vi "Main - ring.vi"() -> ()   [LabVIEW 2024]
doc: "This small application is only a proof of concept. When we have parameters or user data inside an application that could be modified (by the user) at run time, it is important that those changes are 'memorized' when the application is shut down. The next time the application is started it should keep the last configuration made. This is what this application does.\n\nEvery time the user changes the FP data, the changes are saved in the .ini file. If the user closes the application, the FP data is already saved in the .ini configuration file. The next time it is turned on, the data will be loaded again.\n\nIf the user modifies any tag or sector name, or any key name (or its value) in the configuration file (and saves these changes) at run time, the Update button updates this information in the FP of the application, it is the data of the gray fields. This may not be useful in a real application."
uses:
  controls/UI Data.ctl
  controls/string data.ctl
  controls/ring data.ctl
  support/Message Queue/Enqueue Message (Array).vi
  support/Message Queue/Enqueue Message (Single).vi
  dependencies/read-write config ini string data.vi
  <vilib>/Utility/error.llb/Error Cluster From Error Code.vi
  <vilib>/ErrorRing/Error Ring.xnode
  support/Message Queue/Message Queue.lvlib
  support/User Event - Stop/User Event - Stop.lvlib
panel:
  in  "Ring 4":u16(ring) items=["9k", "12k", "18k", "24k"]
  in  "Ring 3":u16(ring) items=["AB ROS", "INVERTER AG", "INVERTER SAMSUNG"]
  in  "Ring 2":u16(ring) items=["MIDEA", "TCL"]
  in  "Ring 1":u16(ring) items=["LOW", "LOW,MID", "LOW,HIGH", "LOW,TURBO", "LOW,MID,HIGH", "LOW,MID,TURBO", "LOW,HIGH,TURBO", "LOW,MID,HIGH,TURBO"]
  out "Display value":string
  in  "Exit":bool
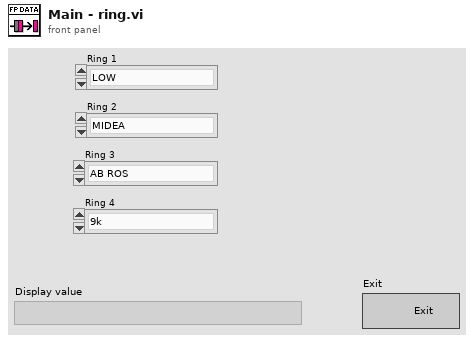
[diagram p1: front panel]
types:
  T1 = typedef "UI Data.ctl" = cluster{"Data Display Ref":refnum<vi>, "Exit Button Ref":refnum<vi>, "user ring data":T2, "ring opts":T2, "Ring Ref":refnum<vi>[], "ring data":T3}
  T2 = typedef "string data.ctl" = cluster{"sectors":string[][], "key names":string[], "values":string[]}
  T3 = typedef "ring data.ctl" = cluster{"option data":string[][]}
  T4 = typedef "Message Queue.lvlib/All Message Queues.ctl" = cluster{"UI":refnum<queue>}
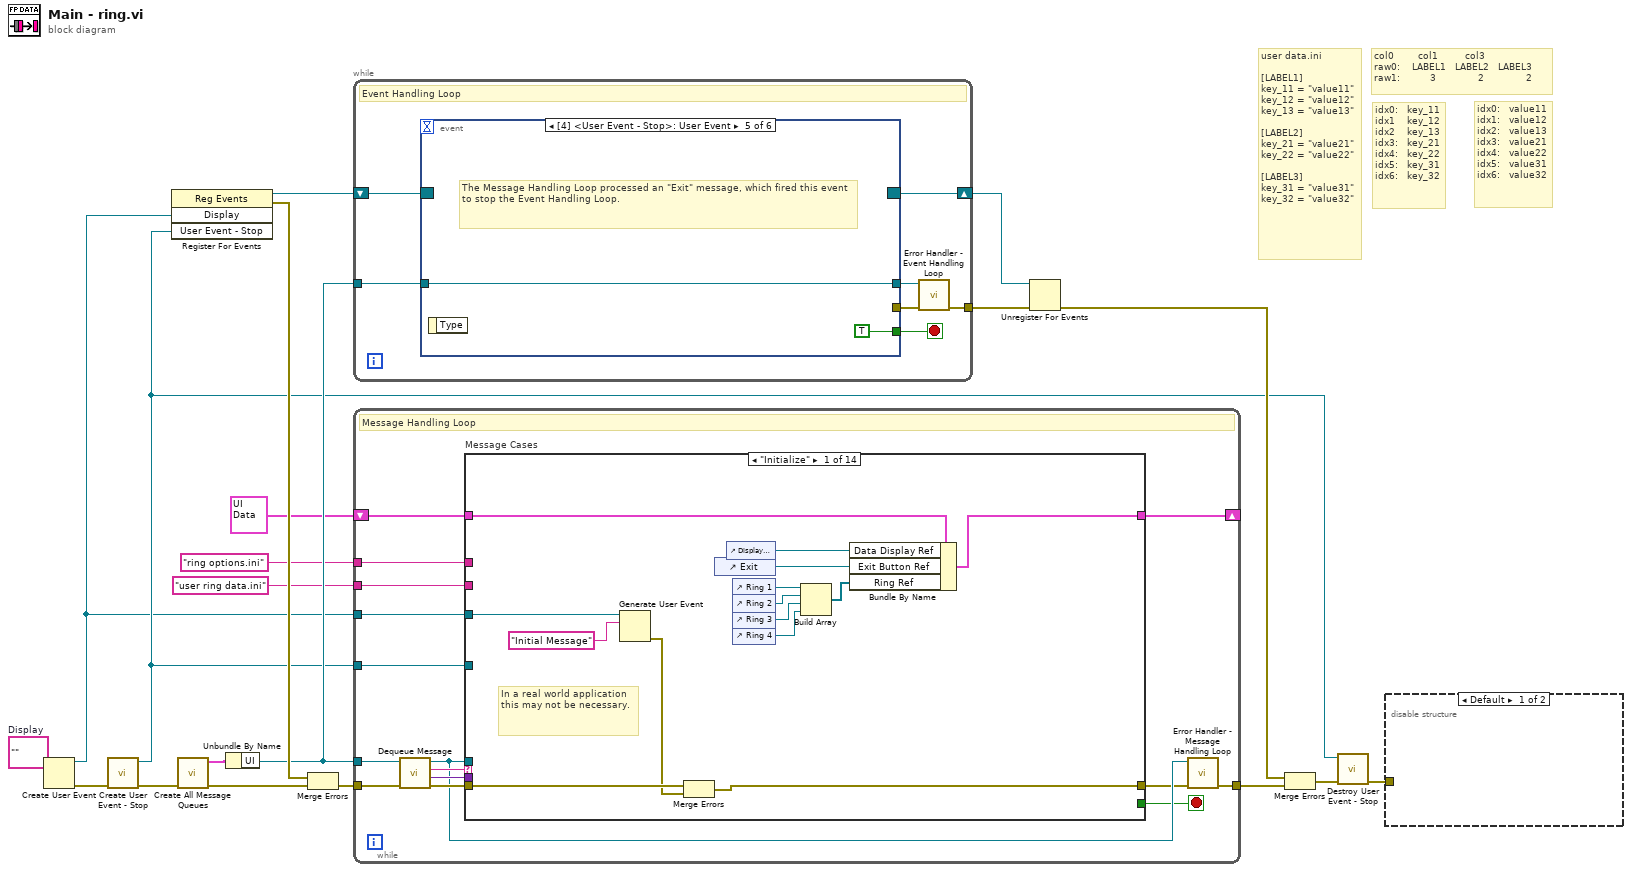
[diagram p0: block diagram]
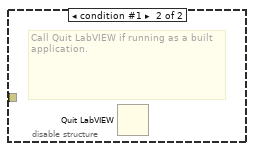
[diagram p2: hidden frame]
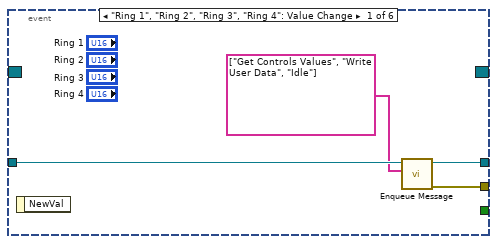
[diagram p3: hidden frame]
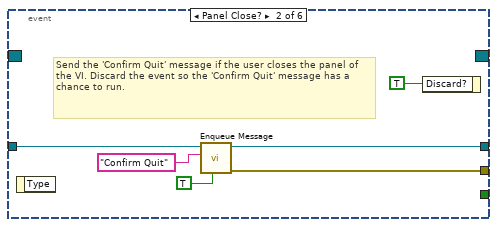
[diagram p4: hidden frame]
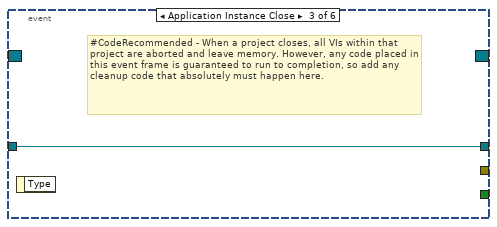
[diagram p5: hidden frame]
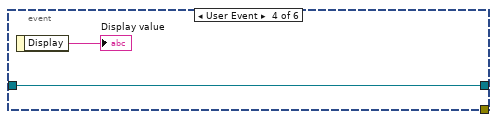
[diagram p6: hidden frame]
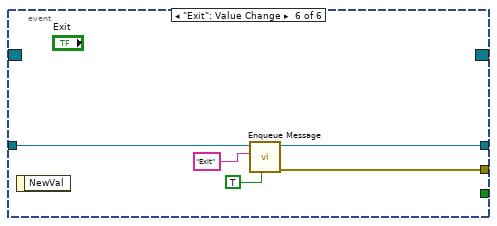
[diagram p7: hidden frame]
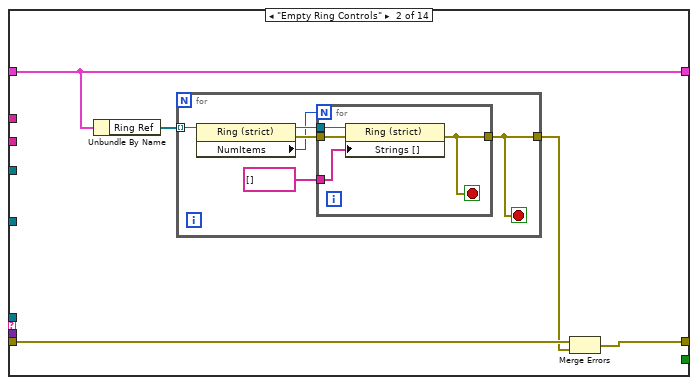
[diagram p8: hidden frame]
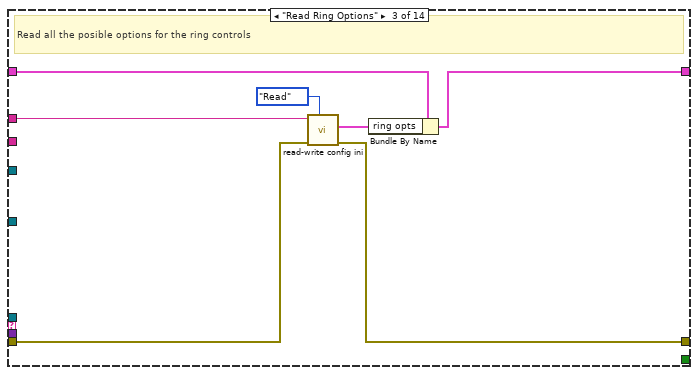
[diagram p9: hidden frame]
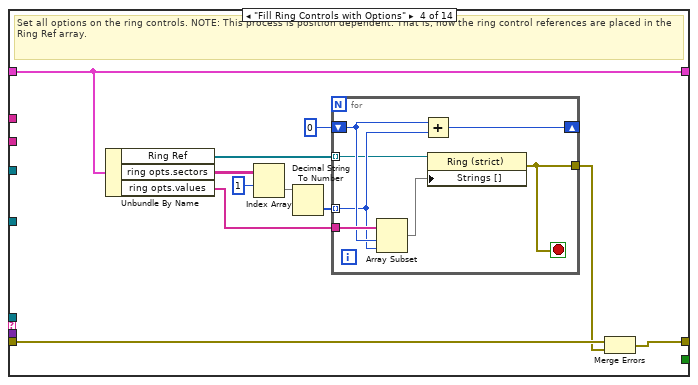
[diagram p10: hidden frame]
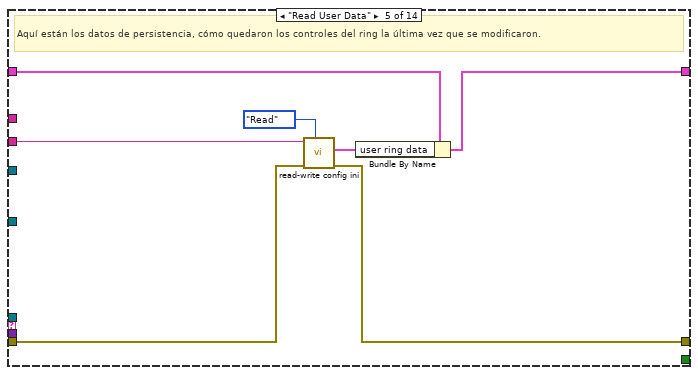
[diagram p11: hidden frame]
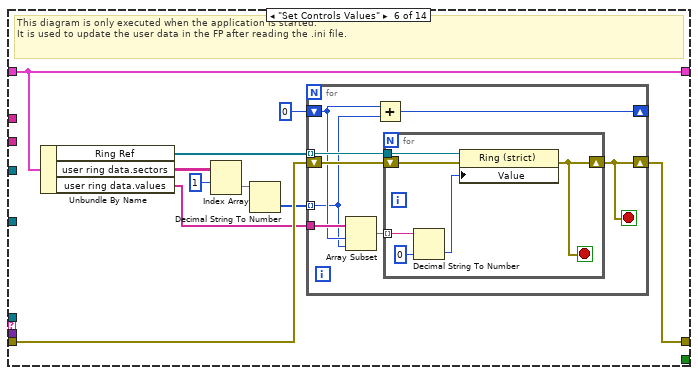
[diagram p12: hidden frame]
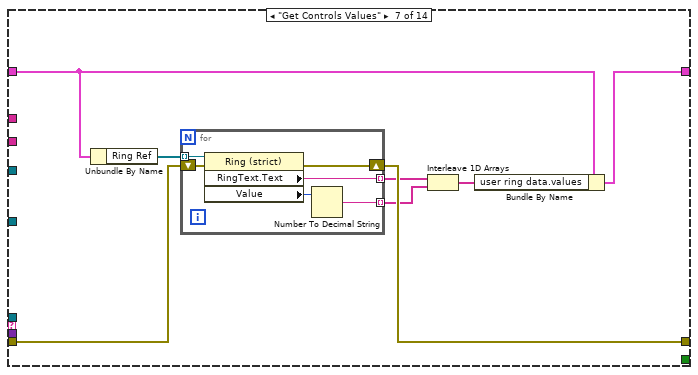
[diagram p13: hidden frame]
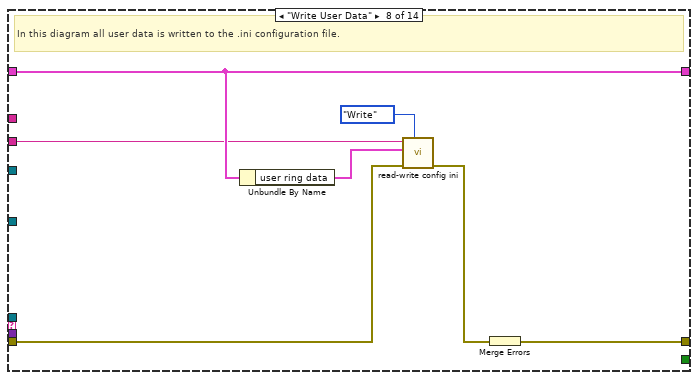
[diagram p14: hidden frame]
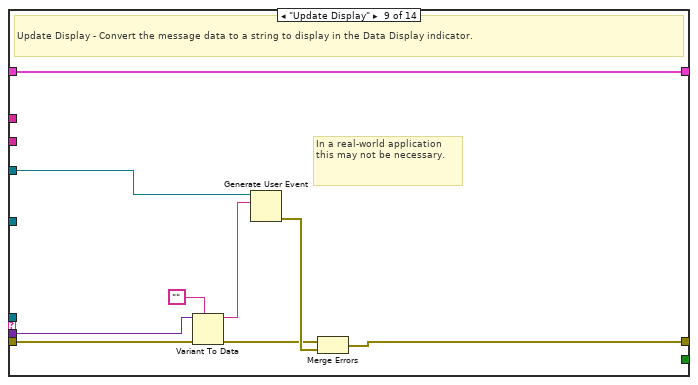
[diagram p15: hidden frame]
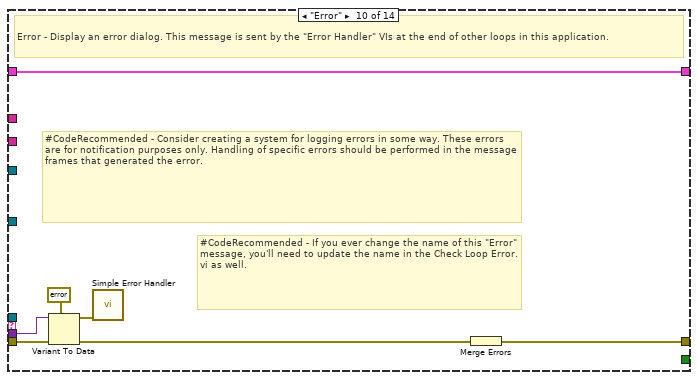
[diagram p16: hidden frame]
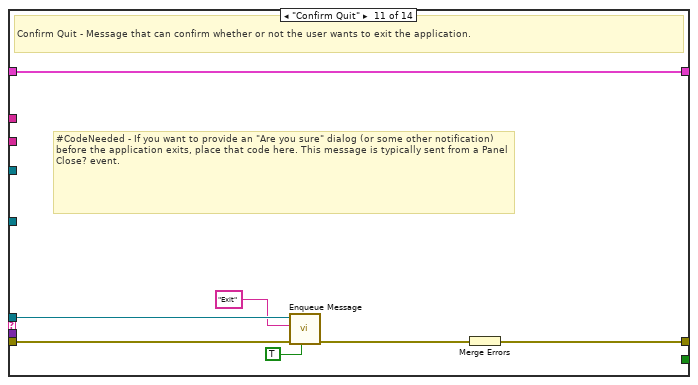
[diagram p17: hidden frame]
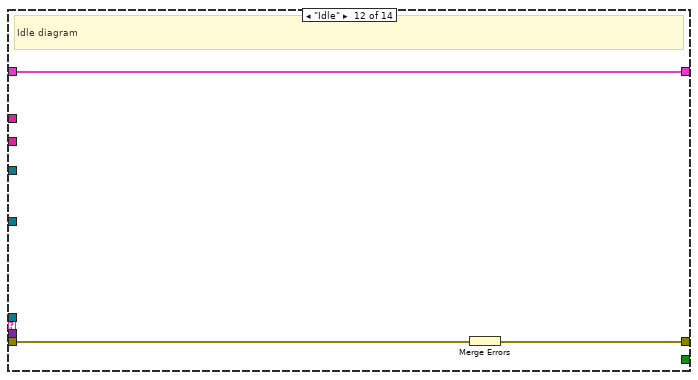
[diagram p18: hidden frame]
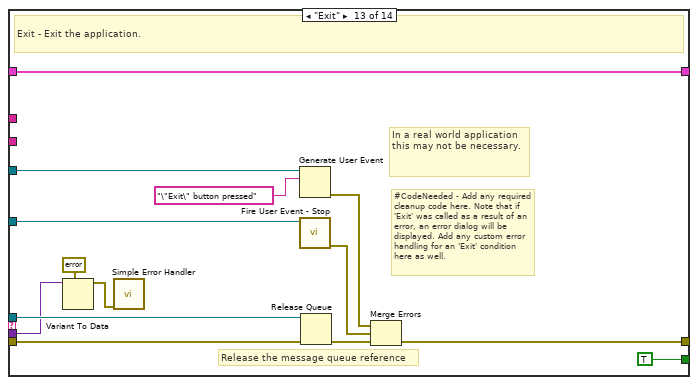
[diagram p19: hidden frame]
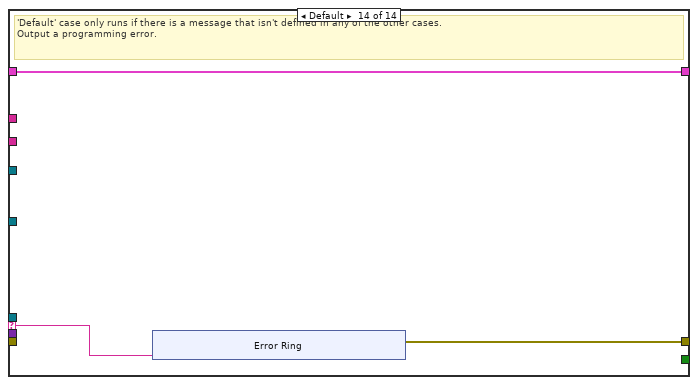
[diagram p20: hidden frame]
diagram:
  w5 = ""  # Display
  # "user data.ini\n\n[LABEL1]\nkey_11 = \"value11\"\nkey_12 = \"value12\"\nkey_13 = \"value13\"\n\n[LABEL2]\nkey_21 = \"value21\"\nkey_22 = \"value22\"\n\n[LABEL3]\nkey_31 = \"value31\"\nkey_32 = \"value32\""
  # "idx0:   value11\nidx1:   value12\nidx2:   value13\nidx3:   value21\nidx4:   value22\nidx5:   value31\nidx6:   value32"
  # "idx0:   key_11\nidx1    key_12\nidx2    key_13\nidx3:   key_21\nidx4:   key_22\nidx5:   key_31\nidx6:   key_32"
  # "col0        col1         col3   \nraw0:    LABEL1   LABEL2   LABEL3\nraw1:          3              2              2"
  n1 = Create User Event(user event datatype=w5) -> (user event=w3:refnum<user-event>, error out=w6:errorcluster)  [unwired: 1 in]
  n2 = call "Create User Event - Stop.vi"("error in (no error)"=w6) -> ("error out"=w15:errorcluster, "User Event - Stop"=w4:refnum<user-event>)  [unwired: 9 in]
  n3 = register-events(w3, w4) -> (reference out=w8:refnum<event-registration>, error out=w20:errorcluster)  [unwired: 2 in]
  n4 = call "Create All Message Queues.vi"("error in (no error)"=w15) -> ("error out"=w19:errorcluster, "Message Queues out"=w18:T4)  [unwired: 9 in]
  n5 = Unbundle By Name(w18) -> ("UI"=w16:refnum<queue>)
  n6 = Merge Errors(w20, w19) -> (w7:errorcluster)
  n7 = while {
    tunnel: w16 -> [w27]
    shift-right: [w25] -> w12
    shift-left: w8 -> [w26]
    tunnel: [w21] -> w9
    stop <- w23 stop-if-true
    # "Event Handling Loop"
    n8 = event shown="[4] <User Event - Stop>: User Event" {
      selector: w26 -> [_ _ _ _ _ _]
      dyn-events: [_ _ _ _ _ _] -> w25
      timeout: _ -> [_ _ _ _ _ _]
      tunnel: [_ _ _ _ TRUE ("Discard?") _] -> w23
      tunnel: w27 -> [w31 w36 w38 w40 w42 w47]
      tunnel: [w29 w35 _ _ _ w46] -> w24
      tunnel: [w30 w34 w38 w40 w42 w45] -> w22
      event "Ring 1", "Ring 2", "Ring 3", "Ring 4": Value Change {
        n9 = event-data() -> ()  [unwired: 1 in, 1 out]
        n10 = call-poly "Enqueue Message.vi"("Message Array"=string[] ["Get Controls Values", "Write User Data", "Idle"], "Message Queue"=w31) -> ("error out"=w29:errorcluster, "dup Message Queue"=w30:refnum<queue>)  [unwired: 8 in]
      }
      event Panel Close? {
        # "Send the 'Confirm Quit' message if the user closes the panel of the VI. Discard the event so the 'Confirm Quit' message has a chance to run."
        n11 = event-data() -> ()  [unwired: 1 in, 1 out]
        n12 = call-poly "Enqueue Message.vi"("Priority Message? (F)"=TRUE, "Message"="Confirm Quit", "Message Queue"=w36) -> ("error out"=w35:errorcluster, "dup Message Queue"=w34:refnum<queue>)  [unwired: 7 in]
        n13 = event-data("Discard?"=TRUE) -> ()  [unwired: 1 in, 1 out]
      }
      event Application Instance Close {
        # "#CodeRecommended - When a project closes, all VIs within that project are aborted and leave memory. However, any code placed in this event frame is guaranteed to run to completion, so add any cleanup code that absolutely must happen here."
        n14 = event-data() -> ()  [unwired: 1 in, 1 out]
      }
      event User Event {
        n15 = event-data() -> ("Display"=→"Display value":string)  [unwired: 1 in]
      }
      event User Event {
        # "The Message Handling Loop processed an \"Exit\" message, which fired this event to stop the Event Handling Loop."
        n16 = event-data() -> ()  [unwired: 1 in, 1 out]
      }
      event "Exit": Value Change {
        n17 = event-data() -> ()  [unwired: 1 in, 1 out]
        n18 = call-poly "Enqueue Message.vi"("Priority Message? (F)"=TRUE, "Message"="Exit", "Message Queue"=w47) -> ("error out"=w46:errorcluster, "dup Message Queue"=w45:refnum<queue>)  [unwired: 7 in]
      }
    }
    n19 = call "Error Handler - Event Handling Loop.vi"("error in (no error)"=w24, "Message Queue"=w22) -> ("dup error in"=w21:errorcluster)  [unwired: 8 in, 1 out]
  }
  n20 = while {
    tunnel: w16 -> [w56]
    shift-right: [w51] -> _
    shift-left: T1 {"Data Display Ref"=refnum, "Exit Button Ref"=refnum, "user ring data"={"sectors"=[], "key names"=[], "values"=[]}, "ring opts"={"sectors"=[], "key names"=[], "values"=[]}, "Ring Ref"=[], "ring data"={"option data"=[]}} ("Data Cluster") -> [w62]
    tunnel: w4 -> [w61]
    tunnel: w7 -> [w60]
    tunnel: [w54] -> w17
    tunnel: w3 -> [w52]
    tunnel: "user ring data.ini" -> [w50]
    tunnel: "ring options.ini" -> [w48]
    stop <- w49 stop-if-true
    # "Message Handling Loop"
    n21 = call "Dequeue Message.vi"("error in (no error)"=w60, "Message Queue"=w56) -> ("error out"=w59:errorcluster, "Message Data"=w57:variant, "Message"=w58:string, "dup Message Queue"=w55:refnum<queue>)  [unwired: 6 in]
    n22 = case "Message Cases" shown="\"Initialize\"" w58 {
      selector: w58 -> [_ _ _ _ _ _ _ _ _ _ _ _ _ w209]
      tunnel: w55 -> [_ _ _ _ _ _ _ _ _ _ w187 _ w208 _]
      tunnel: w59 -> [w72 w81 w96 w109 w119 w133 w154 w162 w172 w184 w191 w194 w201 _]
      tunnel: [w69 w78 w95 w100 w118 w124 w153 w163 w176 w178 w189 w192 w204 w210] -> w53
      tunnel: w62 -> [w76 w80 w94 w108 w123 w132 w150 w168 w177 w183 w190 w193 w207 w211]
      tunnel: [w75 w80 w92 w108 w122 w132 w148 w168 w177 w183 w190 w193 w207 w211] -> w51
      tunnel: [_ _ _ _ _ _ _ _ _ _ _ _ TRUE _] -> w49
      tunnel: w57 -> [_ _ _ _ _ _ _ _ w173 w182 _ _ w198 _]
      tunnel: w61 -> [_ _ _ _ _ _ _ _ _ _ _ _ w203 _]
      tunnel: w52 -> [w71 _ _ _ _ _ _ _ w175 _ _ _ w196 _]
      tunnel: w50 -> [_ _ _ _ w121 _ _ w167 _ _ _ _ _ _]
      tunnel: w48 -> [_ _ w98 _ _ _ _ _ _ _ _ _ _ _]
      frame "Initialize" {
        # "In a real world application this may not be necessary."
        n23 = Generate User Event(user event=w71, event data cluster="Initial Message" ("Initial Message")) -> (error out=w68:errorcluster)  [unwired: 2 in, 1 out]
        n24 = Merge Errors(w72, w68) -> (w69:errorcluster)
        n25 = control-ref of="Exit"() -> (w73:refnum<vi>)
        n26 = control-ref of="Display value"() -> (w74:refnum<vi>)
        n27 = control-ref of="Ring 1"() -> (w67:refnum<vi>)
        n28 = control-ref of="Ring 2"() -> (w66:refnum<vi>)
        n29 = control-ref of="Ring 3"() -> (w65:refnum<vi>)
        n30 = control-ref of="Ring 4"() -> (w64:refnum<vi>)
        n31 = Build Array(w67, w66, w65, w64) -> (w63:refnum<vi>[])
        n32 = Bundle By Name(cluster=w76, "Data Display Ref"=w74, "Exit Button Ref"=w73, "Ring Ref"=w63) -> (w75:T1)
      }
      frame "Empty Ring Controls" {
        n33 = Unbundle By Name(w80) -> ("Ring Ref"=w79:refnum<vi>[])
        n34 = for {
          tunnel: w79 -> [w86] mode=indexing
          tunnel: [w87] -> w77
          stop <- w87 stop-if-true
          n35 = property class="Ring (strict)"(reference=w86) -> (reference out=w85:refnum<vi>, error out=w84:errorcluster, "NumItems"=w83:u32)  [unwired: 1 in]
          n36 = for {
            N: w83 -> [_]
            tunnel: [w91] -> w87
            tunnel: w85 -> [w90]
            tunnel: w84 -> [w89]
            tunnel: string[] [] -> [w88]
            stop <- w91 stop-if-true
            n37 = property class="Ring (strict)"(reference=w90, error in=w89, "Strings []"=w88) -> (error out=w91:errorcluster)  [unwired: 1 out]
          }
        }
        n38 = Merge Errors(w81, w77) -> (w78:errorcluster)
      }
      frame "Read Ring Options" {
        # "Read all the posible options for the ring controls"
        n39 = call-poly "read-write config ini.vi"("Function"=enum16{"Read", "Write"}."Read", "error in (no error)"=w96, "file name"=w98) -> ("error out"=w95:errorcluster, "user data out"=w93:T2)  [unwired: 7 in]
        n40 = Bundle By Name(cluster=w94, "ring opts"=w93) -> (w92:T1)
      }
      frame "Fill Ring Controls with Options" {
        # "Set all options on the ring controls. NOTE: This process is position dependent. That is, how the ring control references are placed in the Ring Ref array."
        n41 = Unbundle By Name(w108) -> ("Ring Ref"=w101:refnum<vi>[], "ring opts.sectors"=w107:string[][], "ring opts.values"=w102:string[])
        n42 = Index Array(array=w107, index (row)=1) -> (element=w105:string[])  [unwired: 1 in]
        n43 = Decimal String To Number(string=w105) -> (number=w104:i32[])  [unwired: 2 in, 1 out]
        n44 = for {
          tunnel: w104 -> [w113] mode=indexing
          shift-right: [w116] -> _
          shift-left: 0 -> [w114]
          tunnel: w102 -> [w115]
          tunnel: w101 -> [w112] mode=indexing
          tunnel: [w110] -> w99
          stop <- w110 stop-if-true
          n45 = Array Subset(array=w115, index=w114, length=w113) -> (w111:string[])
          n46 = Add(x=w114, y=w113) -> (x+y=w116:i32)
          n47 = property class="Ring (strict)"(reference=w112, "Strings []"=w111) -> (error out=w110:errorcluster)  [unwired: 1 in, 1 out]
        }
        n48 = Merge Errors(w109, w99) -> (w100:errorcluster)
      }
      frame "Read User Data" {
        # "Aquí están los datos de persistencia, cómo quedaron los controles del ring la última vez que se modificaron."
        n49 = call-poly "read-write config ini.vi"("Function"=enum16{"Read", "Write"}."Read", "error in (no error)"=w119, "file name"=w121) -> ("error out"=w118:errorcluster, "user data out"=w117:T2)  [unwired: 7 in]
        n50 = Bundle By Name(cluster=w123, "user ring data"=w117) -> (w122:T1)
      }
      frame "Set Controls Values" {
        # "This diagram is only executed when the application is started.\nIt is used to update the user data in the FP after reading the .ini file."
        n51 = Unbundle By Name(w132) -> ("Ring Ref"=w131:refnum<vi>[], "user ring data.sectors"=w128:string[][], "user ring data.values"=w126:string[])
        n52 = Index Array(array=w128, index (row)=1) -> (element=w129:string[])  [unwired: 1 in]
        n53 = Decimal String To Number(string=w129) -> (number=w127:i32[])  [unwired: 2 in, 1 out]
        n54 = for {
          tunnel: w131 -> [w141] mode=indexing
          shift-right: [w139] -> w124
          shift-left: w133 -> [w140]
          tunnel: w127 -> [w135] mode=indexing
          tunnel: w126 -> [w137]
          shift-right: [w138] -> _
          shift-left: 0 -> [w136]
          stop <- w139 stop-if-true
          n55 = Array Subset(array=w137, index=w136, length=w135) -> (w134:string[])
          n56 = Add(x=w136, y=w135) -> (x+y=w138:i32)
          n57 = for {
            tunnel: w141 -> [w147]
            tunnel: w134 -> [w145] mode=indexing
            shift-right: [w142] -> w139
            shift-left: w140 -> [w146]
            stop <- w142 stop-if-true
            n58 = Decimal String To Number(string=w145, default (0L)=u16 0 ("default (0 I32)")) -> (number=w143:u16)  [unwired: 1 in, 1 out]
            n59 = property class="Ring (strict)"(reference=w147, error in=w146, "Value"=w143) -> (error out=w142:errorcluster)  [unwired: 1 out]
          }
        }
      }
      frame "Get Controls Values" {
        n60 = Unbundle By Name(w150) -> ("Ring Ref"=w155:refnum<vi>[])
        n61 = for {
          tunnel: w155 -> [w161] mode=indexing
          tunnel: [w159] -> w152 mode=indexing
          tunnel: [w158] -> w151 mode=indexing
          shift-right: [w157] -> w153
          shift-left: w154 -> [w156]
          n62 = property class="Ring (strict)"(reference=w161, error in=w156) -> (error out=w157:errorcluster, "RingText.Text"=w159:string, "Value"=w160:u16)  [unwired: 1 out]
          n63 = Number To Decimal String(number=w160) -> (decimal integer string=w158:string)  [unwired: 1 in]
        }
        n64 = Interleave 1D Arrays(w152, w151) -> (w149:string[])
        n65 = Bundle By Name(cluster=w150, "user ring data.values"=w149) -> (w148:T1)
      }
      frame "Write User Data" {
        # "In this diagram all user data is written to the .ini configuration file."
        n66 = Unbundle By Name(w168) -> ("user ring data"=w166:T2)
        n67 = call-poly "read-write config ini.vi"("Function"=enum16{"Read", "Write"}."Write", "error in (no error)"=w162, "user data in"=w166, "file name"=w167) -> ("error out"=w164:errorcluster)  [unwired: 6 in, 1 out]
        n68 = Merge Errors(w164) -> (w163:errorcluster)
      }
      frame "Update Display" {
        # "In a real-world application this may not be necessary."
        # "Update Display - Convert the message data to a string to display in the Data Display indicator."
        n69 = Variant To Data(error in=w172, type="", Variant=w173) -> (data=w169:string, error out=w171:errorcluster)
        n70 = Generate User Event(user event=w175, event data cluster=w169) -> (error out=w174:errorcluster)  [unwired: 2 in, 1 out]
        n71 = Merge Errors(w171, w174) -> (w176:errorcluster)
      }
      frame "Error" {
        # "#CodeRecommended - If you ever change the name of this \"Error\" message, you'll need to update the name in the Check Loop Error.vi as well."
        # "#CodeRecommended - Consider creating a system for logging errors in some way. These errors are for notification purposes only. Handling of specific errors should be performed in the message frames that generated the error."
        # "Error - Display an error dialog. This message is sent by the \"Error Handler\" VIs at the end of other loops in this application."
        n72 = Variant To Data(error in=w184, type=errorcluster {"status"=FALSE, "code"=0, "source"=""} ("error constant"), Variant=w182) -> (data=w180:errorcluster, error out=w179:errorcluster)
        n73 = call <vilib>:"Simple Error Handler.vi"("error in (no error)"=w180) -> ()  [unwired: 4 in, 5 out]
        n74 = Merge Errors(w179) -> (w178:errorcluster)
      }
      frame "Confirm Quit" {
        # "#CodeNeeded - If you want to provide an \"Are you sure\" dialog (or some other notification) before the application exits, place that code here. This message is typically sent from a Panel Close? event."
        # "Confirm Quit - Message that can confirm whether or not the user wants to exit the application."
        n75 = call-poly "Enqueue Message.vi"("Priority Message? (F)"=TRUE, "error in (no error)"=w191, "Message"="Exit", "Message Queue"=w187) -> ("error out"=w188:errorcluster)  [unwired: 6 in, 1 out]
        n76 = Merge Errors(w188) -> (w189:errorcluster)
      }
      frame "Idle" {
        # "Idle diagram"
        n77 = Merge Errors(w194) -> (w192:errorcluster)
      }
      frame "Exit" {
        # "In a real world application this may not be necessary."
        # "Release the message queue reference"
        # "#CodeNeeded - Add any required cleanup code here. Note that if 'Exit' was called as a result of an error, an error dialog will be displayed. Add any custom error handling for an 'Exit' condition here as well."
        # "Exit - Exit the application."
        n78 = Variant To Data(type=errorcluster {"status"=FALSE, "code"=0, "source"=""} ("error constant"), Variant=w198) -> (data=w199:errorcluster)  [unwired: 1 in, 1 out]
        n79 = call <vilib>:"Simple Error Handler.vi"("error in (no error)"=w199) -> ()  [unwired: 4 in, 5 out]
        n80 = Generate User Event(user event=w196, event data cluster="\"Exit\" button pressed" ("Initial Message")) -> (error out=w195:errorcluster)  [unwired: 2 in, 1 out]
        n81 = call "Fire User Event - Stop.vi"("User Event - Stop"=w203) -> ("error out"=w202:errorcluster)  [unwired: 10 in]
        n82 = Release Queue(queue=w208, error in (no error)=w201) -> (error out=w205:errorcluster)  [unwired: 1 in, 2 out]
        n83 = Merge Errors(w195, w202, w205) -> (w204:errorcluster)
      }
      frame Default {
        # "'Default' case only runs if there is a message that isn't defined in any of the other cases.\nOutput a programming error."
        n84 = xnode "Error Ring"("parameter 0"=w209) -> ("error out"=w210:errorcluster)
      }
    }
    n85 = call "Error Handler - Message Handling Loop.vi"("error in (no error)"=w53, "Message Queue"=w55) -> ("dup error in"=w54:errorcluster)  [unwired: 8 in, 1 out]
  }
  n86 = Unregister For Events(event registration refnum=w12, error in=w9) -> (error out=w13:errorcluster)
  n87 = Merge Errors(w13, w17) -> (w14:errorcluster)
  n88 = call "Destroy User Event - Stop.vi"("error in (no error)"=w14, "User Event - Stop"=w4) -> ("error out"=w10:errorcluster)  [unwired: 9 in]
  n89 = disable-structure shown="Default" {
    disable-tunnel: w10 -> [_ _]
    frame condition #0 (active) {
    }
    frame condition #1 {
      # "Call Quit LabVIEW if running as a built application."
      n90 = Quit LabVIEW() -> ()  [unwired: 1 in]
    }
  }
